vi "DataCom.vi"() -> ()   [LabVIEW 2020, in "ModBus Serial Master.lvlib"]
uses:
  ModBus Serial Master.lvlib
  DriverCommon/MB Modbus Command.ctl
  DriverCommon/Swap.ctl
  DriverCommon.lvlib
  ModBusCommon.lvlib
panel:
  out "MB_CMD_Out":T1[](array[typedef]) {"Function Code" items=["Read Coils"=1, "Read Discrete Inputs"=2, "Read Holding Registers"=3, "Read Input Registers"=4, "Write Single Coil"=5, "Write Single Register"=6, "Read Exception Status"=7, "Write Multiple Coils"=15, "Write Multiple Registers"=16]}
  out "deleted portion":T1={"Function Code"=1, "Starting Address"=0, "Quantity"=0, "Data"=[], "Discrete"=[], "Index of Tags"=[]} {"Function Code" items=["Read Coils"=1, "Read Discrete Inputs"=2, "Read Holding Registers"=3, "Read Input Registers"=4, "Write Single Coil"=5, "Write Single Register"=6, "Read Exception Status"=7, "Write Multiple Coils"=15, "Write Multiple Registers"=16]}
  out "Registers":cluster{"Registers":u16[], "Discrete":bool[]}
  in  "Device Index":i32
  in  "POLL":bool
  in  "Swap":T2
  in  "SDC":string
  in  "Index":i32 caption="SDC Index"
  in  "Interval":u32=50
  in  "Serial":refnum<visa-resource-name> caption="Serial Interface"
  in  "Mode":enum16{"RTU", "ASCII"}(ring)
  in  "Communication Status":string
  out "Communication Information":string[][](table)
  out "Command Interval":u32
  in  "Timeout":u32=5000
  out "Device Scanning Cycle":u32
  in  "Modbus Command":T1[](array[typedef]) {"Function Code" items=["Read Coils"=1, "Read Discrete Inputs"=2, "Read Holding Registers"=3, "Read Input Registers"=4, "Write Single Coil"=5, "Write Single Register"=6, "Read Exception Status"=7, "Write Multiple Coils"=15, "Write Multiple Registers"=16]}
  in  "SlaveAddress":string="1" caption="Slave Address"
  in  "Stop":bool
  # "ModBus Serial Master Driver"
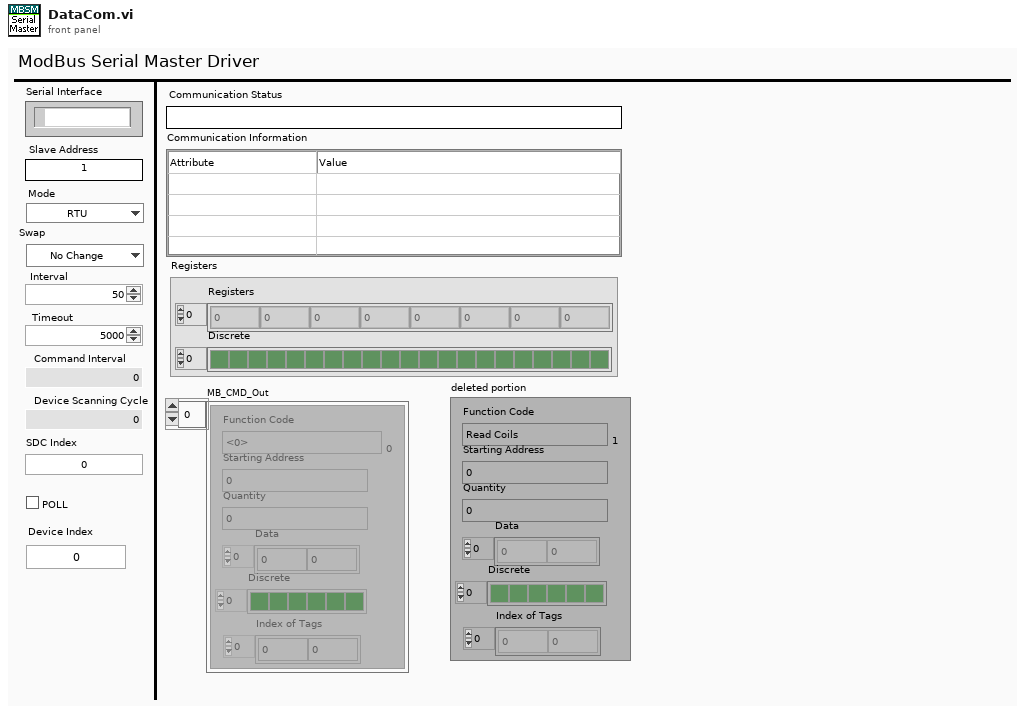
[diagram p1: front panel]
types:
  T1 = typedef "DriverCommon.lvlib/MB Modbus Command.ctl" = cluster{"Function Code":u8, "Starting Address":u16, "Quantity":u16, "Data":u16[], "Discrete":bool[], "Index of Tags":i32[]}
  T2 = typedef "DriverCommon.lvlib/Swap.ctl" = enum16{"No Change", "Swap"}
  T3 = cluster{"Mode":enum16{"RTU", "ASCII"}, "Slave Address":u8}
  T4 = cluster{"notifier out":refnum<notifier>, "POLL":bool}
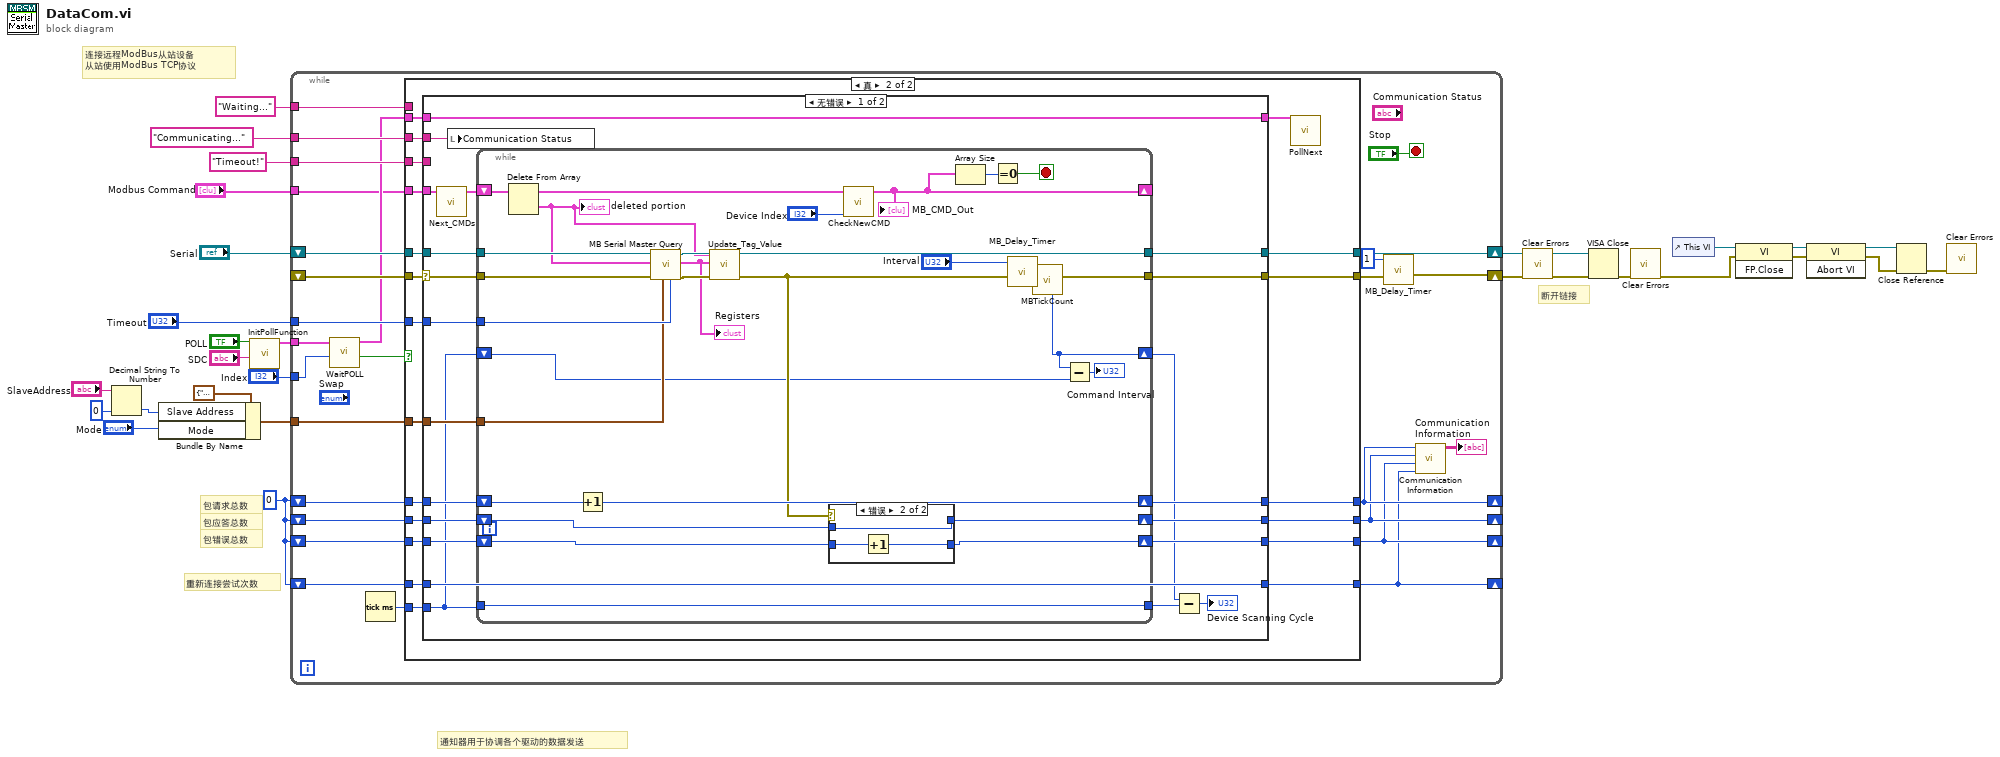
[diagram p0: block diagram]
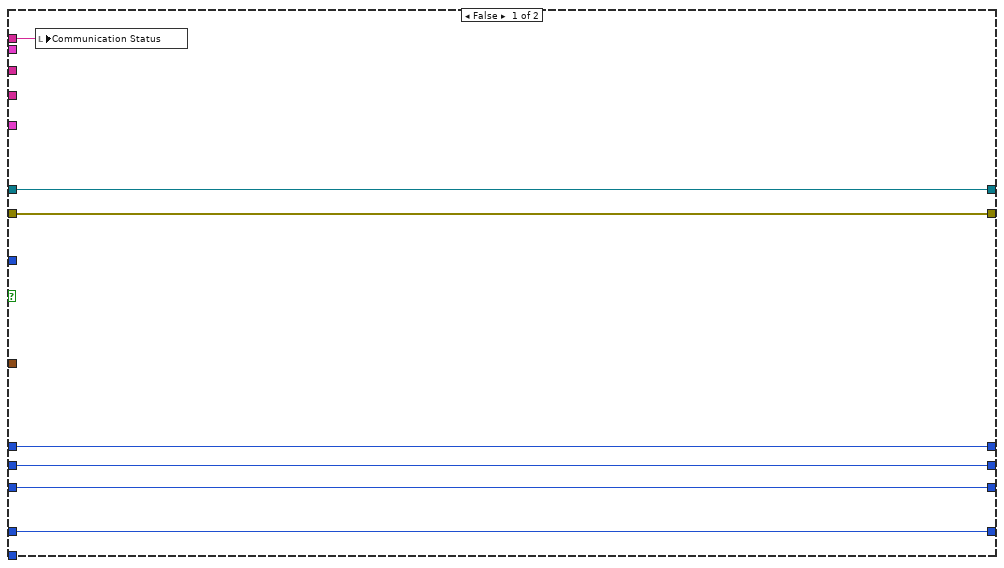
[diagram p2: hidden frame]
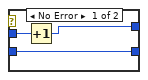
[diagram p3: hidden frame]
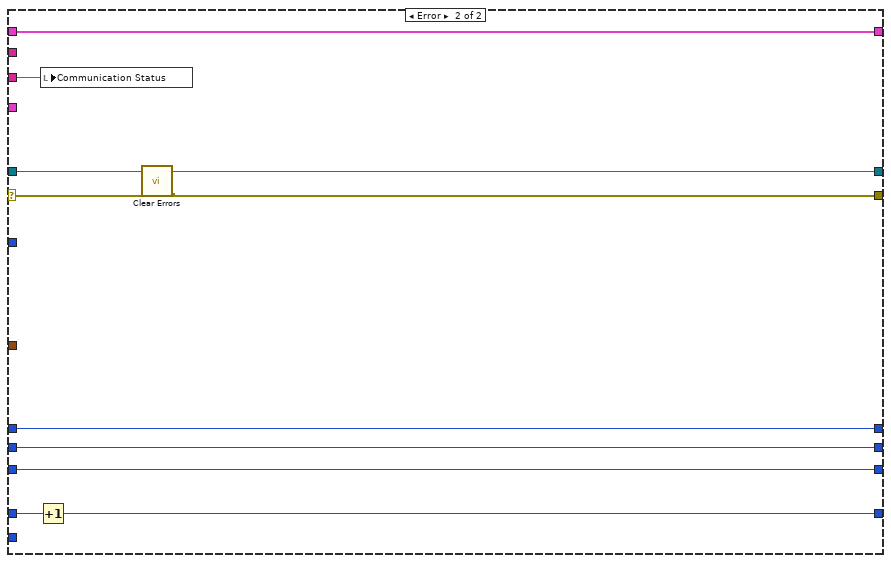
[diagram p4: hidden frame]
diagram:
  w23 = 0
  # "通知器用于协调各个驱动的数据发送"
  # "重新连接尝试次数"
  # "包错误总数"
  # "包应答总数"
  # "包请求总数"
  # "断开链接"
  # "连接远程ModBus从站设备\n从站使用ModBus TCP协议"
  n1 = Decimal String To Number(string="SlaveAddress", default (0L)=u8 0 ("default (0 I32)")) -> (number=w19:u8)  [unwired: 1 in, 1 out]
  n2 = Bundle By Name(cluster=T3 {"Mode"=enum."RTU", "Slave Address"=0} ("Serial Parameters"), "Slave Address"=w19, "Mode"="Mode") -> (w21:T3)
  n3 = call "InitPollFunction.vi"("SDC"="SDC", "POLL"="POLL") -> ("notifier out"=w7:T4)  [unwired: 9 in]
  n4 = while {
    shift-right: [w37] -> w12
    shift-left: _ -> [w52]
    tunnel: "Timeout" -> [w51]
    tunnel: "Timeout!" ("Communication Status") -> [w50]
    tunnel: "Communicating..." ("Communication Status") -> [w49]
    shift-right: [w43] -> _
    shift-left: w23 -> [w47]
    shift-right: [w42] -> _
    shift-left: w23 -> [w46]
    shift-right: [w41] -> _
    shift-left: w23 -> [w45]
    shift-right: [w40] -> _
    shift-left: w23 -> [w48]
    shift-right: [w54] -> w13
    shift-left: "Serial" -> [w55]
    tunnel: w21 -> [w39]
    tunnel: w7 -> [w33]
    tunnel: "Index" -> [w31]
    tunnel: "Waiting..." ("Communication Status") -> [w35]
    tunnel: "Modbus Command" -> [w29]
    stop <- "Stop" stop-if-true
    n5 = call "WaitPOLL.vi"("Index"=w31, "notifier In"=w33) -> ("Polled"=w32:bool, "notifier out"=w30:T4)  [unwired: 8 in]
    n6 = Tick Count (ms)() -> (millisecond timer value=w34:u32)
    n7 = case shown="真" w32 {
      tunnel: w55 -> [w62 w82]
      tunnel: [w62 w81] -> w54
      tunnel: [w61 w80] -> w38
      tunnel: w52 -> [w61 w79]
      tunnel: w51 -> [_ w78]
      tunnel: w50 -> [_ w77]
      tunnel: w49 -> [_ w76]
      tunnel: w48 -> [w57 w75]
      tunnel: w47 -> [w60 w74]
      tunnel: w46 -> [w59 w73]
      tunnel: w45 -> [w58 w72]
      tunnel: [w60 w71] -> w43
      tunnel: [w59 w70] -> w42
      tunnel: [w58 w69] -> w41
      tunnel: [w57 w68] -> w40
      tunnel: w39 -> [_ w67]
      tunnel: w30 -> [_ w66]
      tunnel: w35 -> [w56 _]
      tunnel: w34 -> [_ w65]
      tunnel: w29 -> [_ w63]
      frame False {
        n8 = local write "Communication Status"(w56) -> ()
      }
      frame True {
        n9 = case shown="无错误" w79 {
          selector: w79 -> [w100 w140]
          tunnel: w82 -> [w103 w138]
          tunnel: [w102 w138] -> w81
          tunnel: [w101 w139] -> w80
          tunnel: w78 -> [w99 _]
          tunnel: w77 -> [_ w146]
          tunnel: w76 -> [w98 _]
          tunnel: [w97 w144] -> w68
          tunnel: w75 -> [w97 w145]
          tunnel: [w95 w143] -> w71
          tunnel: w74 -> [w94 w143]
          tunnel: [w93 w142] -> w70
          tunnel: w73 -> [w92 w142]
          tunnel: [w91 w141] -> w69
          tunnel: w72 -> [w90 w141]
          tunnel: w67 -> [w89 _]
          tunnel: [w88 w137] -> w64
          tunnel: w66 -> [w88 w137]
          tunnel: w65 -> [w84 _]
          tunnel: w63 -> [w83 _]
          frame No Error {
            n10 = call "Next_CMDs.vi"("MBCMDs"=w83) -> ("MBCMD Out"=w96:T1[])  [unwired: 10 in]
            n11 = local write "Communication Status"(w98) -> ()
            n12 = while {
              tunnel: w103 -> [w130]
              tunnel: [w129] -> w102
              tunnel: w100 -> [w128]
              tunnel: [w114] -> w101
              tunnel: w99 -> [w127]
              shift-right: [w112] -> w87
              shift-left: w84 -> [w113]
              tunnel: w89 -> [w119]
              shift-right: [w125] -> w95
              shift-left: w94 -> [w124]
              shift-right: [w123] -> w93
              shift-left: w92 -> [w122]
              shift-right: [w121] -> w91
              shift-left: w90 -> [w120]
              tunnel: [w116] -> w86
              tunnel: w84 -> [w116]
              shift-right: [w106] -> _
              shift-left: w96 -> [w110]
              stop <- w105 stop-if-true
              n13 = Delete From Array(array=w110) -> (deleted portion=w109:T1, array with subset deleted=w104:T1[])  [unwired: 2 in]
              "deleted portion" <- w109
              n14 = Increment(x=w124) -> (x+1=w125:i32)
              n15 = call "MB Serial Master Query.vi"("Timeout"=w127, "Serial Parameters"=w119, "error in (no error)"=w128, "Modbus Command"=w109, "VISA resource name"=w130) -> ("error out"=w118:errorcluster, "Registers"=w111:cluster{"Registers":u16[], "Discrete":bool[]}, "VISA resource name out"=w129:refnum<visa-resource-name>)  [unwired: 1 in, 3 out]
              "Registers" <- w111
              n16 = call "Update_Tag_Value.vi"("Registers"=w111, "MB Command"=w109) -> ()  [unwired: 10 in]
              n17 = case shown="错误" w118 {
                tunnel: w122 -> [w133 w136]
                tunnel: [w132 w136] -> w123
                tunnel: [w131 w134] -> w121
                tunnel: w120 -> [w131 w135]
                frame No Error {
                  n18 = Increment(x=w133) -> (x+1=w132:i32)
                }
                frame Error {
                  n19 = Increment(x=w135) -> (x+1=w134:i32)
                }
              }
              n20 = call "CheckNewCMD.vi"("DeviceIndex"="Device Index", "MB_CMD_In"=w104) -> ("MB_CMD_Out"=w106:T1[])  [unwired: 9 in]
              "MB_CMD_Out" <- w106
              n21 = Array Size(array=w106) -> (size(s)=w107:i32)
              n22 = Equal To 0?(x=w107) -> (x = 0?=w105:bool)
              n23 = call "MB_Delay_Timer.vi"("error in (no error)"=w118, "Delay_Time(ms)"="Interval") -> ("error out"=w115:errorcluster)  [unwired: 9 in]
              n24 = call "MBTickCount.vi"("error in (no error)"=w115) -> ("error out"=w114:errorcluster, "millisecond timer value"=w112:u32)  [unwired: 9 in]
              n25 = Subtract(x=w112, y=w113) -> (x-y=→"Command Interval":u32)
            }
            n26 = Subtract(x=w87, y=w86) -> (x-y=→"Device Scanning Cycle":u32)
          }
          frame Error {
            n27 = Increment(x=w145) -> (x+1=w144:i32)
            n28 = local write "Communication Status"(w146) -> ()
            n29 = call <vilib>:"Clear Errors.vi"("error in (no error)"=w140) -> ("error out"=w139:errorcluster)  [unwired: 5 in, 1 out]
          }
        }
        n30 = call "PollNext.vi"("notifier In"=w64) -> ()  [unwired: 11 in]
      }
    }
    n31 = call "MB_Delay_Timer.vi"("error in (no error)"=w38, "Delay_Time(ms)"=u32 1) -> ("error out"=w37:errorcluster)  [unwired: 9 in]
    n32 = call "Communication Information.vi"("Total Interrupt"=w40, "Total Error Answer"=w41, "Total Answer"=w42, "Total Request"=w43) -> ("output array"=→"Communication Information":string[][])  [unwired: 7 in]
  }
  n33 = call <vilib>:"Clear Errors.vi"("error in (no error)"=w12) -> ("error out"=w11:errorcluster)  [unwired: 5 in, 1 out]
  n34 = VISA Close(VISA resource name=w13, error in (no error)=w11) -> (error out=w10:errorcluster)
  n35 = call <vilib>:"Clear Errors.vi"("error in (no error)"=w10) -> ("error out"=w5:errorcluster)  [unwired: 5 in, 1 out]
  n36 = control-ref of="This VI"() -> (w6:refnum<vi>)
  n37 = invoke class="VI" method="FP.Close"(reference=w6, error in=w5) -> (reference out=w28:refnum<vi>, error out=w27:errorcluster)  [unwired: 1 in, 1 out]
  n38 = invoke class="VI" method="Abort VI"(reference=w28, error in=w27) -> (reference out=w4:refnum<vi>, error out=w3:errorcluster)  [unwired: 1 in, 1 out]
  n39 = Close Reference(reference=w4, error in (no error)=w3) -> (error out=w2:errorcluster)
  n40 = call <vilib>:"Clear Errors.vi"("error in (no error)"=w2) -> ()  [unwired: 5 in, 2 out]
